vi "DS_write_wrapper.vi"(0 "Connection In":string, 2 "ms timeout (0)":i32, 3 "rawData":variant, 5 "error in":errorcluster) -> (14 "connection out":string, 16 "timed out":bool, 19 "error out":errorcluster)   [LabVIEW 2012, in "HGF_SV.lvlib"]
doc: "Wrapper for Datasocket write VI to avoid LabVIEW crash. LabVIEW has a bug opening a network shared variable with datasocket in a VI with dynamic terminals. This wrapper prevents that because it has no dynamic terminals :)"
uses:
  HGF_SV.lvlib
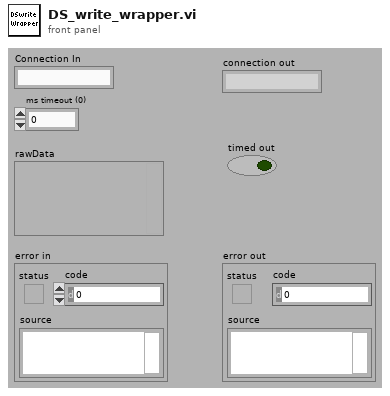
[diagram p1: front panel]
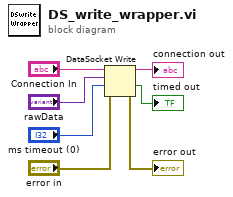
[diagram p0: block diagram]
diagram:
  n1 = DataSocket Write(8:"error in", 9:"ms timeout (0)", 10:"rawData", 11:"Connection In") -> (0:→"error out":errorcluster, 1:→"timed out":bool, 3:→"connection out":string)
